vi "DSF.Engine.Transfer.Get Intermediate Buffer.vi"(11 "Transfer in":refnum<class "DSF.Engine.Transfer.lvclass">) -> (2 "DBL Buffer":refnum<class "DSF.Engine.Pointer.DBL.lvclass">, 3 "Transfer out":refnum<class "DSF.Engine.Transfer.lvclass">)   [LabVIEW 2017, in "DSF.Engine.lvlib" / "DSF.Engine.Transfer.lvclass"]
uses:
  DSF.Engine.Transfer.lvclass
  Pointer/DSF.Engine.Pointer.DBL.lvclass
  DSF.Engine.Transfer.lvclass/DSF.Engine.Transfer.ctl
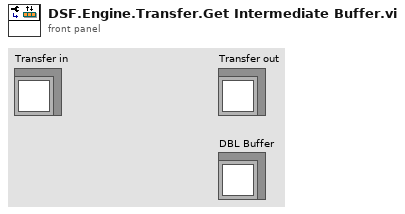
[diagram p1: front panel]
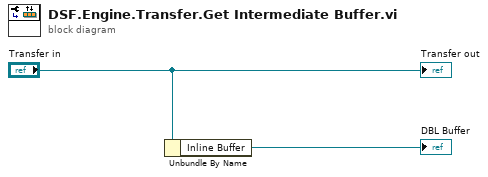
[diagram p0: block diagram]
diagram:
  n1 = Unbundle By Name("Transfer in") -> ("Inline Buffer"=→"DBL Buffer":refnum<class "DSF.Engine.Pointer.DBL.lvclass">)
  "Transfer out" <- "Transfer in"
